vi "Tektronix DPO MSO 2000 4000 Series Acquire Multiple Waveform Example.vi"() -> ()   [LabVIEW 2009]
doc: "This example illustrates how to use autosetup and acquire multiple waveforms from several channels using the following steps:\n\n1. Specify a valid VISA session. \n2. Specify Channel A. \n3. Specify Channel B.\n4. Specify a time-out value for reading waveform.\n5. Run the VI. The graph displays waveforms you acquire."
uses:
  <instrlib>/Tektronix DPO MSO 2000 4000 Series/Public/Data/Read (Multiple Waveforms).vi
  <instrlib>/Tektronix DPO MSO 2000 4000 Series/Tektronix DPO MSO 2000 4000 Series.lvlib
panel:
  in  "Vertical Coupling (1: DC)":u16(ring)=1 items=["AC", "DC", "Ground"]
  in  "Vertical Coupling (1: DC)":u16(ring)=1 items=["AC", "DC", "Ground"]
  in  "Maximum Time (20000ms)":u32=20000
  in  "Channel B (1: Channel 2)":u16(ring)=1 items=["Channel 1", "Channel 2", "Channel 3", "Channel 4", "Math", "Reference 1", "Reference 2", "Reference 3", "Reference 4"]
  in  "Channel A (0: Channel 1)":u16(ring) items=["Channel 1", "Channel 2", "Channel 3", "Channel 4", "Math", "Reference 1", "Reference 2", "Reference 3", "Reference 4"]
  in  "VISA Resource Name":refnum<visa-resource-name>
  out "Waveform Graph":waveform(dbl)[](graph)
  # "(C) 2006 - 2013. National Instruments Corporation. ALL RIGHTS RESERVED."
  # "Channel A"
  # "Channel B"
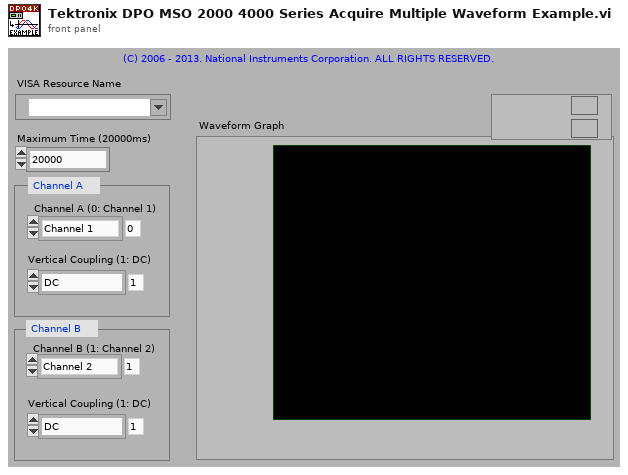
[diagram p1: front panel]
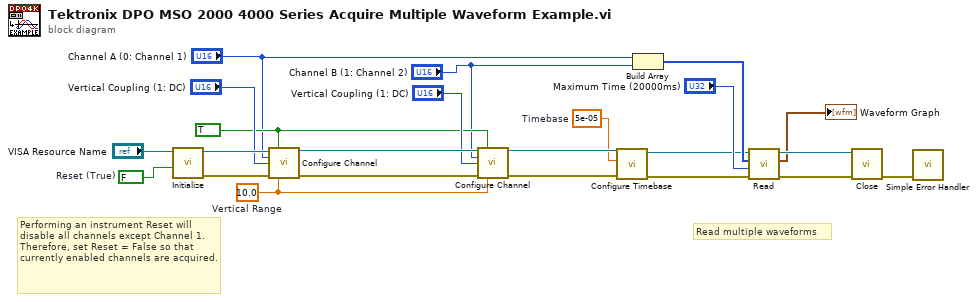
[diagram p0: block diagram]
diagram:
  w5 = 5e-05  # Timebase
  w3 = 10.0  # Vertical Range
  w4 = TRUE ("Enable Channel (T: Enable)")
  w16 = FALSE  # Reset (True)
  # "Performing an instrument Reset will disable all channels except Channel 1. Therefore, set Reset = False so that currently enabled channels are acquired."
  # "Read multiple waveforms"
  n1 = call <instrlib>:"Initialize.vi"("Reset (True)"=w16, "VISA resource name"="VISA Resource Name") -> ("error out"=w14:errorcluster, "VISA resource name out"=w15:refnum<visa-resource-name>)  [unwired: 8 in]
  n2 = call <instrlib>:"Configure Channel.vi"("VISA resource name"=w15, "Enable Channel (T: Enable)"=w4, "Channel (0: Channel 1)"="Channel A (0: Channel 1)", "Vertical Coupling (1: DC)"="Vertical Coupling (1: DC)", "error in (no error)"=w14, "Vertical Range (10.0 V)"=w3) -> ("VISA resource name out"=w13:refnum<visa-resource-name>, "error out"=w12:errorcluster)  [unwired: 8 in]
  n3 = call <instrlib>:"Configure Channel.vi"("VISA resource name"=w13, "Enable Channel (T: Enable)"=w4, "Channel (0: Channel 1)"="Channel B (1: Channel 2)", "Vertical Coupling (1: DC)"="Vertical Coupling (1: DC)", "error in (no error)"=w12, "Vertical Range (10.0 V)"=w3) -> ("VISA resource name out"=w9:refnum<visa-resource-name>, "error out"=w8:errorcluster)  [unwired: 8 in]
  n4 = call <instrlib>:"Configure Timebase.vi"("error in (no error)"=w8, "Timebase (0.0005 s)"=w5, "VISA resource name"=w9) -> ("error out"=w6:errorcluster, "VISA resource name out"=w7:refnum<visa-resource-name>)  [unwired: 7 in]
  n5 = Build Array("Channel A (0: Channel 1)", "Channel B (1: Channel 2)") -> (w22:u16[])
  n6 = call-poly <instrlib>:"Read.vi"("error in (no error)"=w6, "Maximum Time (10000ms)"="Maximum Time (20000ms)", "Channels"=w22, "VISA resource name"=w7) -> ("error out"=w20:errorcluster, "Waveform Data"=→"Waveform Graph":waveform(dbl)[], "VISA resource name out"=w21:refnum<visa-resource-name>)  [unwired: 5 in]
  n7 = call <instrlib>:"Close.vi"("error in (no error)"=w20, "VISA resource name"=w21) -> ("error out"=w18:errorcluster)  [unwired: 9 in]
  n8 = call <vilib>:"Simple Error Handler.vi"("error in (no error)"=w18) -> ()  [unwired: 4 in, 5 out]
